vi "Delay Judge.vi"(8 "error in (no error)":errorcluster caption="Error In", 9 "Delay Time(ms)":u32, 10 "Restart":bool, 11 "Count Time(ms)":u32) -> (0 "error out":errorcluster caption="Error Out", 1 "Count":u32, 2 "Time Out?":bool, 3 "Elapsed time(ms)":u32, 4 "Restart？":bool)   [LabVIEW 2020]
doc: "开发者 ：加油小林哥\n功能 ：此vi用于流程控制中的延时\n输入：\nCount Time(ms) : 每次的计数间隔,单位为ms\nRestart : 是否重新计数\nDelay Time(ms) : 每次经过此vi的延时时间\n输出：\nElapsed Time(ms)：每次计数的延时时间，此时间小于Coumt Time\nTimeout？ ： 是否达到计数时间\nCount ：计数次数\nRestart？ ：是否重新开始计数，两种情况会重新开始计数（1、首次调用此vi；2、Restart置为Ture；）"
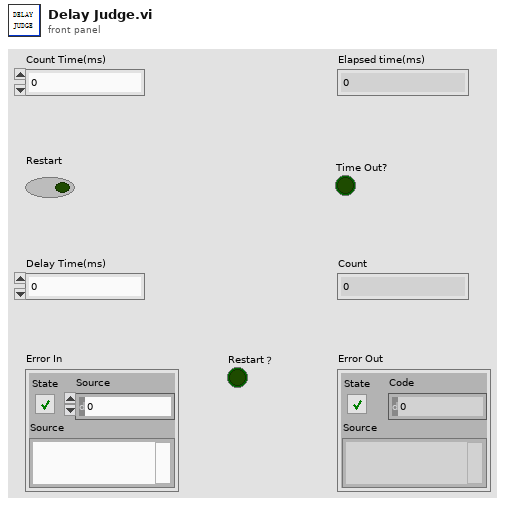
[diagram p1: front panel]
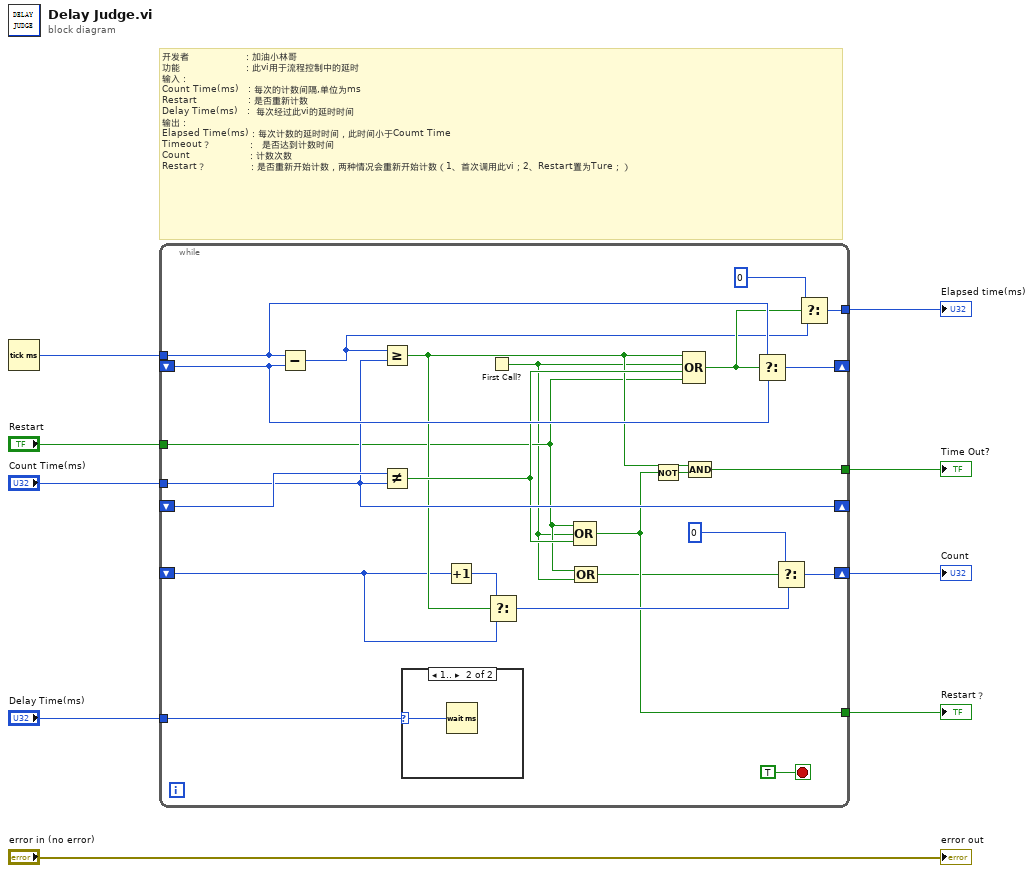
[diagram p0: block diagram]
diagram:
  # "开发者                  ：加油小林哥\n功能                     ：此vi用于流程控制中的延时\n输入：\nCount Time(ms)   : 每次的计数间隔,单位为ms\nRestart                 : 是否重新计数\nDelay Time(ms)   :  每次经过此vi的延时时间\n输出：\nElapsed Time(ms)：每次计数的延时时间，此时间小于Coumt Time\nTimeout？            ：  是否达到计数时间\nCount                   ：计数次数\nRestart？              ：是否重新开始计数，两种情况会重新开始计数（1、首次调用此vi；2、Restart置为Ture；）"
  n1 = Tick Count (ms)() -> (millisecond timer value=w7:u32)
  n2 = while {
    tunnel: w7 -> [w31]
    shift-right: [w33] -> _
    shift-left: _ -> [w30]
    tunnel: "Count Time(ms)" -> [w28]
    tunnel: [w23] -> w8
    shift-right: [w28] -> _
    shift-left: _ -> [w29]
    tunnel: [w27] -> w5
    shift-right: [w20] -> w4
    shift-left: _ -> [w17]
    tunnel: "Delay Time(ms)" -> [w14]
    tunnel: "Restart" -> [w12]
    tunnel: [w13] -> w1
    stop <- TRUE stop-if-true
    n3 = Subtract(x=w31, y=w30) -> (x-y=w24:u32)
    n4 = Greater Or Equal?(x=w24, y=w28) -> (x >= y?=w19:bool)
    n5 = Not Equal?(x=w29, y=w28) -> (x != y?=w22:bool)
    n6 = case shown="1.." w14 {
      selector: w14 -> [_ w34]
      frame 0, Default {
      }
      frame 1.. {
        n7 = Wait (ms)(milliseconds to wait=w34) -> ()  [unwired: 1 out]
      }
    }
    n8 = Increment(x=w17) -> (x+1=w18:u32)
    n9 = First Call?() -> (First Call?: T/F=w11:bool)
    n10 = Select(t=w18, s=w19, f=w17) -> (s? t:f=w16:u32)
    n11 = Compound Arithmetic op=OR ("复合运算")(w12, w11, w22) -> (w13:bool)
    n12 = Compound Arithmetic op=OR ("复合运算")(w12, w11) -> (w10:bool)
    n13 = Not(x=w13) -> (.not. x?=w15:bool)
    n14 = Compound Arithmetic op=OR ("复合运算")(w19, w11, w22, w12) -> (w26:bool)
    n15 = Compound Arithmetic op=AND ("复合运算")(w19, w15) -> (w27:bool)
    n16 = Select(t=w31, s=w26, f=w30) -> (s? t:f=w33:u32)
    n17 = Select(t=u32 0 ("millisecond timer value"), s=w10, f=w16) -> (s? t:f=w20:u32)
    n18 = Select(t=u32 0 ("millisecond timer value"), s=w26, f=w24) -> (s? t:f=w23:u32)
  }
  "Time Out?" <- w5
  "Elapsed time(ms)" <- w8
  "Count" <- w4
  "Restart？" <- w1
  "error out" <- "error in (no error)"
